vi "Program22.vi"() -> ()   [LabVIEW 2020]
panel:
  out "Usuniete elementy":i32[](array[numeric])
  out "Pozostale":i32[](array[numeric])
  out "Tablica":i32[](array[numeric])
  in  "Dlugosc":i32(slide) scale=0.0..10.0
  in  "Index":i32(slide) scale=0.0..10.0
  in  "Ilosc iteracji":i32
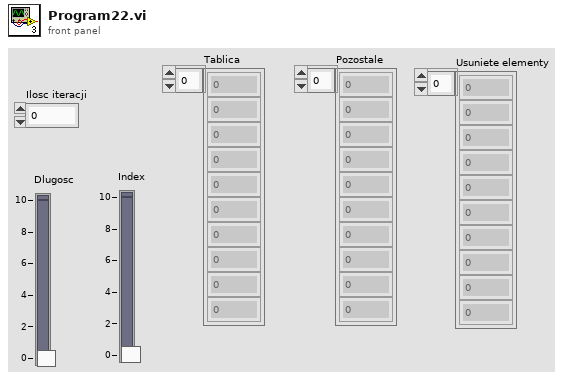
[diagram p1: front panel]
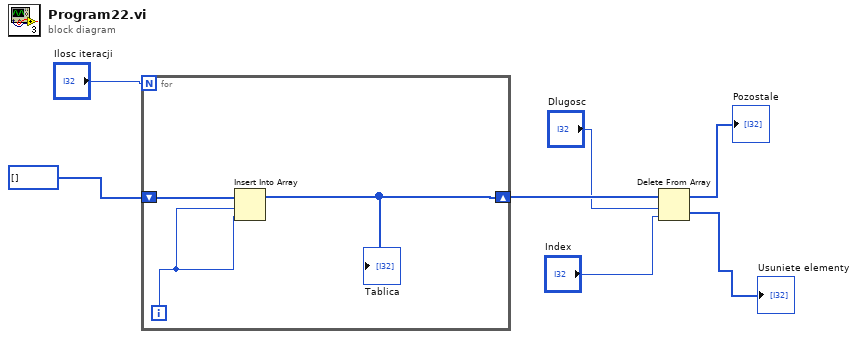
[diagram p0: block diagram]
diagram:
  n1 = for {
    N: "Ilosc iteracji" -> [_]
    shift-right: [w8] -> w5
    shift-left: i32[] [] -> [w9]
    i -> [w10]
    n2 = Insert Into Array(array=w9, index=w10, new element=w10) -> (w8:i32[])
    "Tablica" <- w8
  }
  n3 = Delete From Array(array=w5, length="Dlugosc", index="Index") -> (deleted portion=→"Usuniete elementy":i32[], array with subset deleted=→"Pozostale":i32[])
